vi "classify type.vi"(11 "data type":T1) -> (2 "array?":bool, 3 "numeric?":bool)   [LabVIEW 2013, in "data bus tag description.lvclass"]
uses:
  data bus tag description.lvclass
  Data Type.ctl
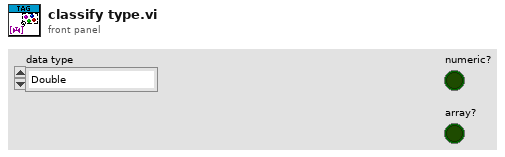
[diagram p1: front panel]
types:
  T1 = typedef "data bus tag description.lvclass/Data Type.ctl" = enum16{"Double", "I64", "Boolean", "Array of Double", "Array of I64", "Variant"}
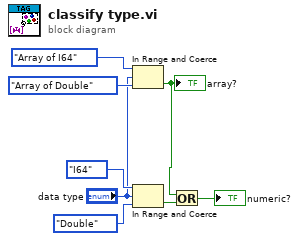
[diagram p0: block diagram]
diagram:
  n1 = In Range and Coerce(upper limit=Data_Type."Array of I64", x="data type", lower limit=Data_Type."Array of Double") -> (In Range?=w1:bool)  [unwired: 1 out]
  "array?" <- w1
  n2 = In Range and Coerce(upper limit=Data_Type."I64", x="data type", lower limit=Data_Type."Double") -> (In Range?=w6:bool)  [unwired: 1 out]
  n3 = Or(x=w1, y=w6) -> (x .or. y?=→"numeric?":bool)
